vi "SEQ Release Queue.vi"(8 "error in (no error)":errorcluster, 11 "Queue Name":string) -> (0 "error out":errorcluster)   [LabVIEW 2019, in "ADLINK Motion Card.lvlib"]
uses:
  ADLINK Motion Card.lvlib
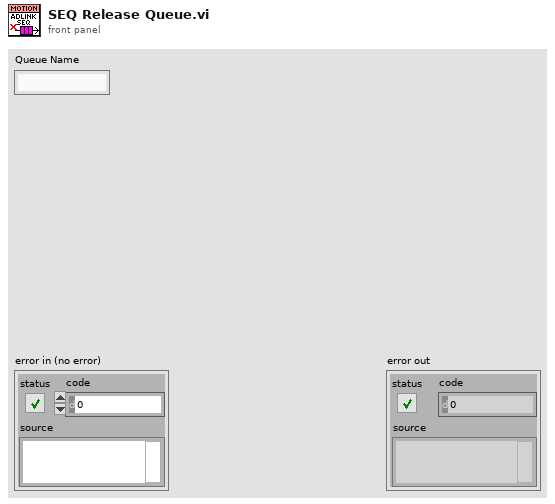
[diagram p1: front panel]
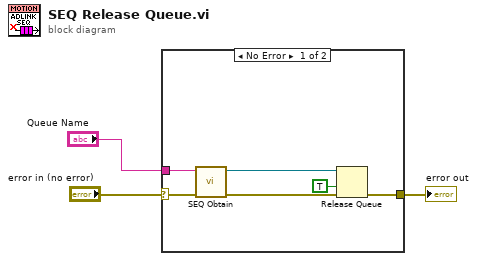
[diagram p0: block diagram]
diagram:
  n1 = case shown="No Error" "error in (no error)" {
    selector: "error in (no error)" -> [w8 w10]
    tunnel: "Queue Name" -> [w9 _]
    tunnel: [w7 w10] -> w1
    frame No Error {
      n2 = call "SEQ Obtain.vi"("error in (no error)"=w8, "Queue Name"=w9) -> ("error out"=w5:errorcluster, "queue out"=w6:refnum<queue>)  [unwired: 8 in]
      n3 = Release Queue(queue=w6, force destroy? (F)=TRUE, error in (no error)=w5) -> (error out=w7:errorcluster)  [unwired: 2 out]
    }
    frame Error {
    }
  }
  "error out" <- w1
